vi "WLAN_be_EVMvi.vi"(5 "Function":T1, 7 "setPower":i32, 8 "error in":errorcluster, 11 "VISA IN":refnum<visa-resource-name>="IQGIG") -> (0 "error out":errorcluster, 1 "EVM":dbl, 2 "Power":dbl, 3 "IDN":string)   [LabVIEW 2023, in "LitePoints.lvlib"]
uses:
  LitePoints.lvlib
  CTL/LitePoint_EVM.ctl
panel:
  out "forREF_PW":string
  out "Response_EVM":string
  out "Response_PW":string
  out "VSA_Ref?":string
  out "VSA?":string
  out "Clean Buffer?":string
  out "setPower?":string
  # "IQgig-5G : TCPIP0::192.168.100.254::hislip0::INSTR"
  # "IQxel-MX : TCPIP0::192.168.100.253::hislip0::INSTR"
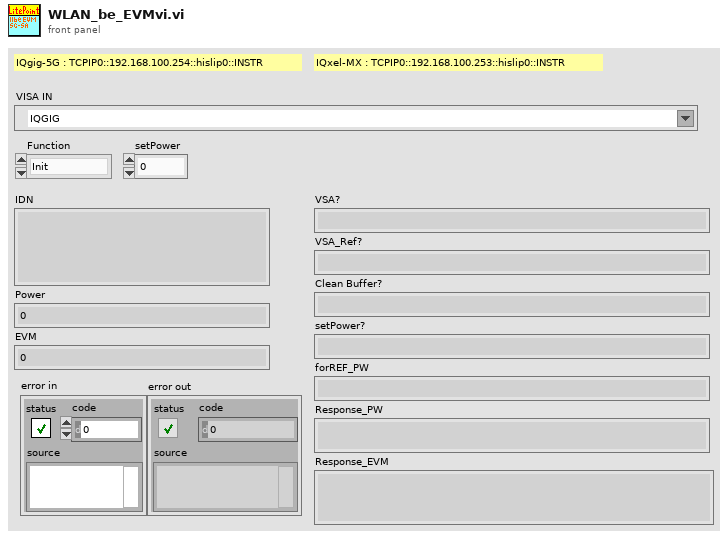
[diagram p1: front panel]
types:
  T1 = typedef "LitePoint_EVM.ctl" = enum16{"Init", "Close", "set_SG", "set_SA", "get_EVM", "byPass", "getPower"}
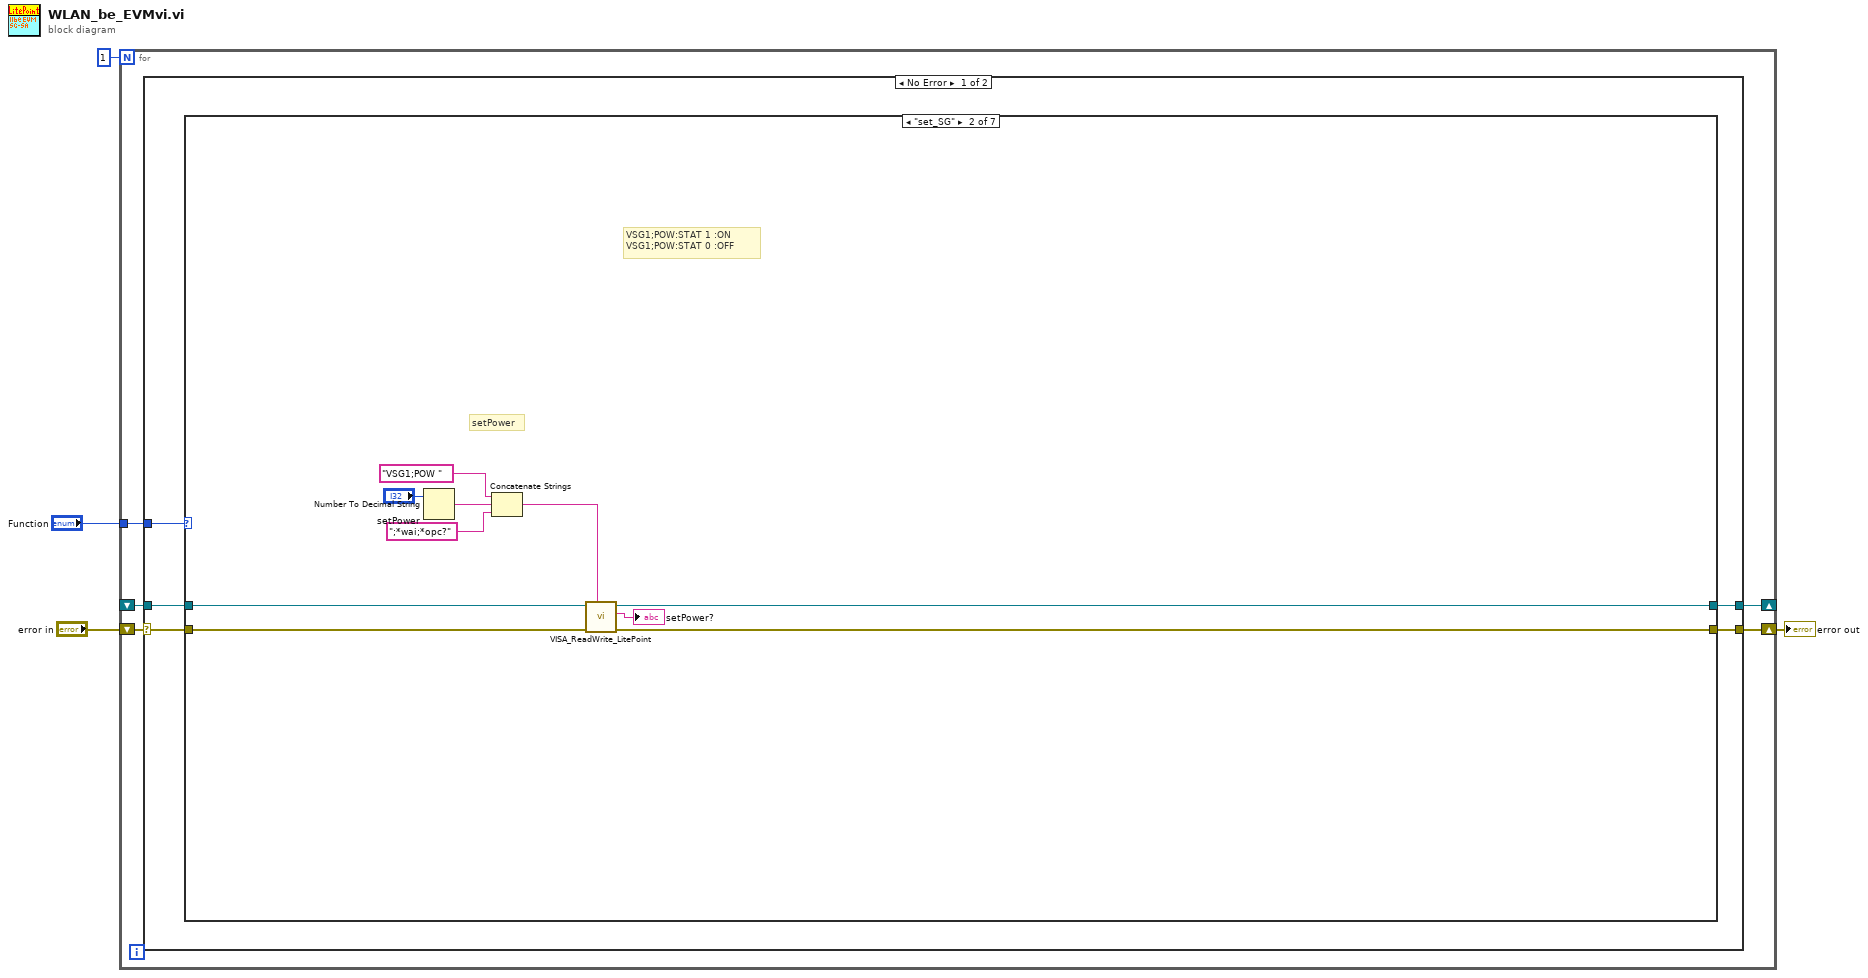
[diagram p0: block diagram]
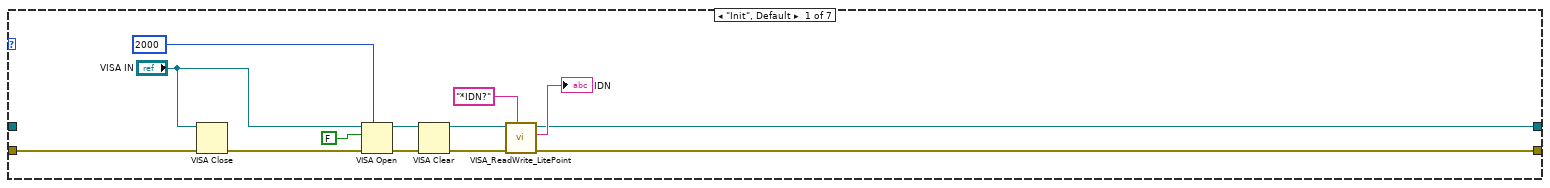
[diagram p2: hidden frame]
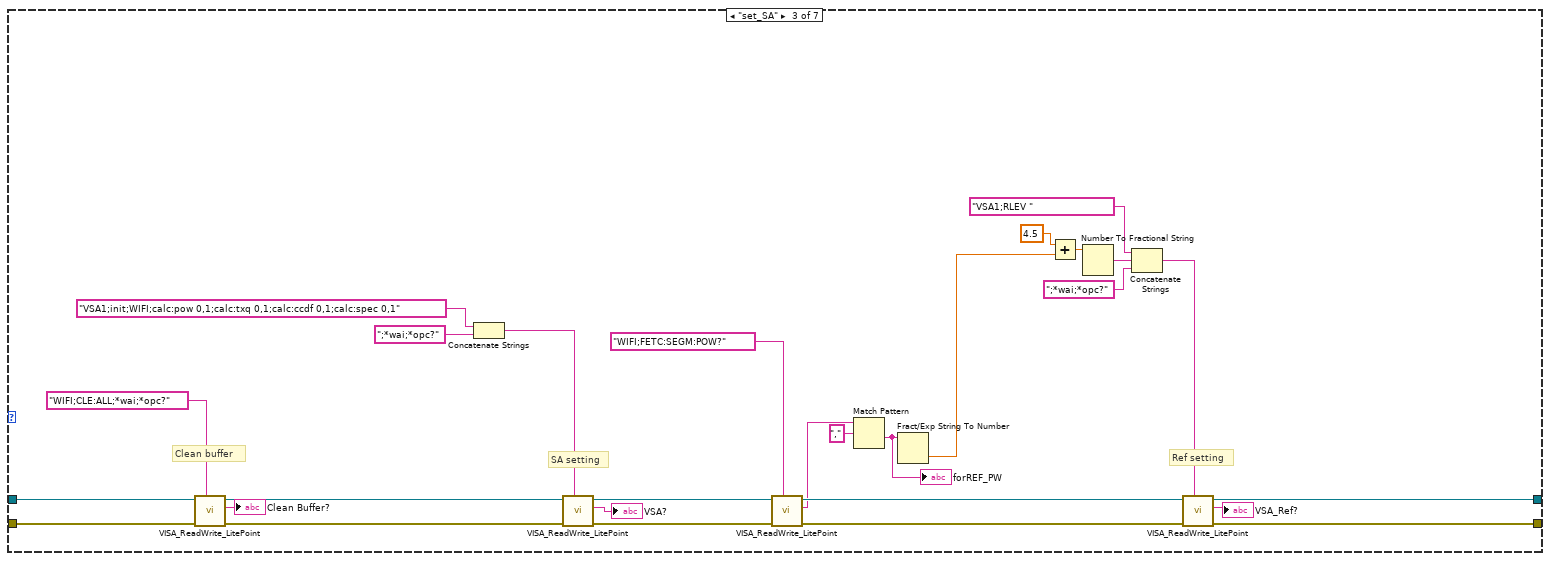
[diagram p3: hidden frame]
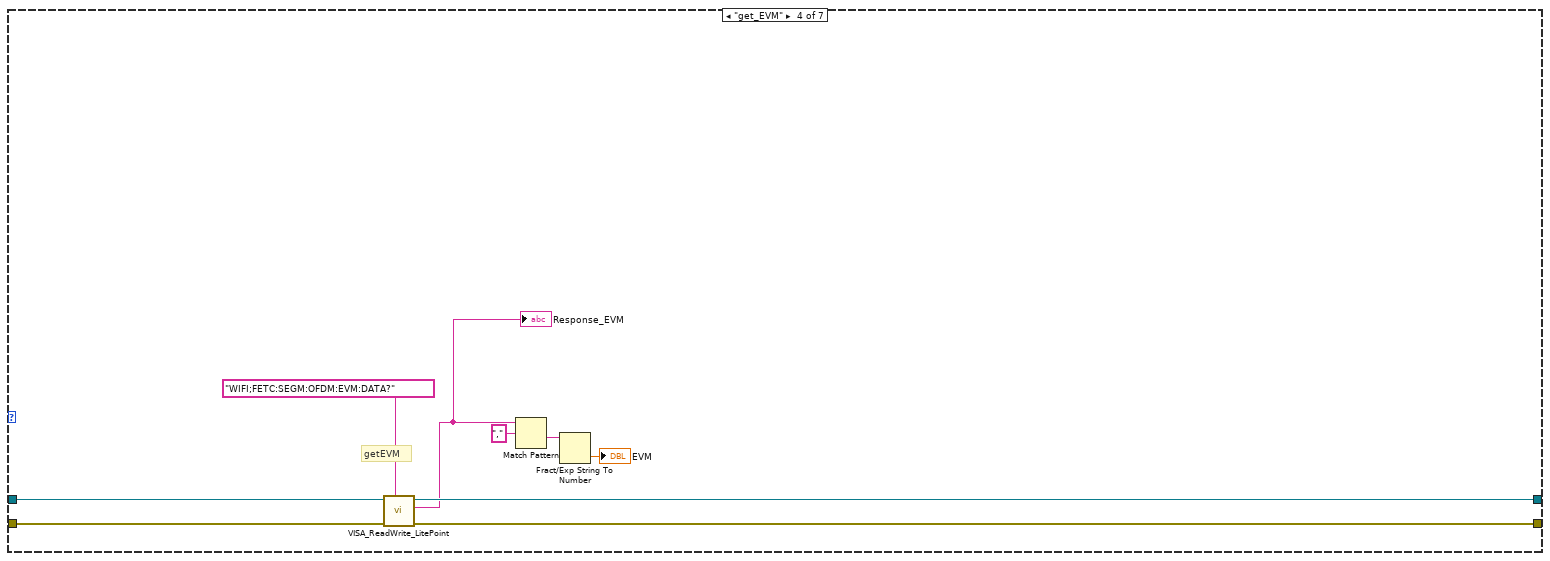
[diagram p4: hidden frame]
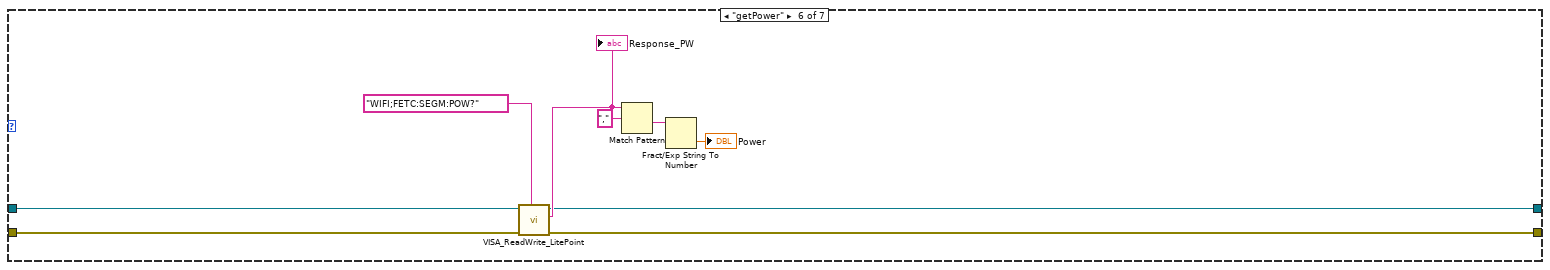
[diagram p6: hidden frame]
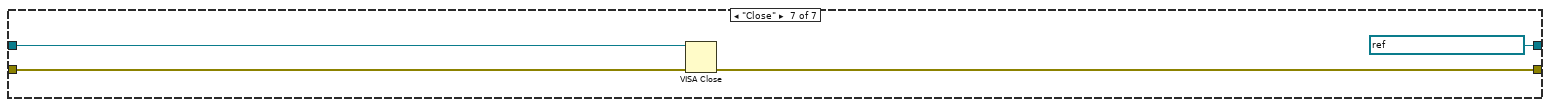
[diagram p7: hidden frame]
diagram:
  n1 = for {
    N: 1 -> [_]
    tunnel: "Function" -> [w7]
    shift-right: [w8] -> w3
    shift-left: "error in" -> [w9]
    shift-right: [w5] -> _
    shift-left: _ -> [w6]
    n2 = case shown="No Error" w9 {
      selector: w9 -> [w13 w91]
      tunnel: [w12 w91] -> w8
      tunnel: w7 -> [w14 _]
      tunnel: w6 -> [w11 w90]
      tunnel: [w10 w90] -> w5
      frame No Error {
        n3 = case shown="\"set_SG\"" w14 {
          tunnel: [w22 w28 w51 w71 w76 w84 w89] -> w12
          tunnel: w13 -> [w17 w32 w65 w74 w76 w85 w88]
          tunnel: w11 -> [_ w33 w64 w73 w75 w79 w87]
          tunnel: [w18 w29 w52 w70 w75 w78 refnum<visa-resource-name> refnum ("VISA out")] -> w10
          frame "Init", Default {
            n4 = VISA Close(VISA resource name="VISA IN", error in (no error)=w17) -> (error out=w16:errorcluster)
            n5 = VISA Open(timeout (0)=u32 2000 ("VISA Open timeout (0)"), duplicate session (F)=FALSE, error in (no error)=w16, VISA resource name="VISA IN") -> (VISA resource name=w24:refnum<visa-resource-name>, error out=w25:errorcluster)  [unwired: 1 in]
            n6 = VISA Clear(VISA resource name=w24, error in (no error)=w25) -> (VISA resource name out=w21:refnum<visa-resource-name>, error out=w23:errorcluster)
            n7 = call "VISA_ReadWrite_LitePoint.vi"("VISA_CMD"="*IDN?", "error in"=w23, "VISA in"=w21) -> ("error out"=w22:errorcluster, "Response"=→"IDN":string, "VISA out"=w18:refnum<visa-resource-name>)  [unwired: 6 in]
          }
          frame "set_SG" {
            # "VSG1;POW:STAT 1 :ON\nVSG1;POW:STAT 0 :OFF"
            # "setPower"
            n8 = Number To Decimal String(number="setPower") -> (decimal integer string=w37:string)  [unwired: 1 in]
            n9 = Concatenate Strings("VSG1;POW " ("write buffer"), w37, ";*wai;*opc?" ("write buffer")) -> (w31:string)
            n10 = call "VISA_ReadWrite_LitePoint.vi"("VISA_CMD"=w31, "error in"=w32, "VISA in"=w33) -> ("error out"=w28:errorcluster, "Response"=→"setPower?":string, "VISA out"=w29:refnum<visa-resource-name>)  [unwired: 6 in]
          }
          frame "set_SA" {
            # "Ref setting"
            # "SA setting"
            # "Clean buffer"
            n11 = call "VISA_ReadWrite_LitePoint.vi"("VISA_CMD"="WIFI;CLE:ALL;*wai;*opc?" ("write buffer"), "error in"=w65, "VISA in"=w64) -> ("error out"=w57:errorcluster, "Response"=→"Clean Buffer?":string, "VISA out"=w58:refnum<visa-resource-name>)  [unwired: 6 in]
            n12 = Concatenate Strings("VSA1;init;WIFI;calc:pow 0,1;calc:txq 0,1;calc:ccdf 0,1;calc:spec 0,1" ("write buffer"), ";*wai;*opc?" ("write buffer")) -> (w59:string)
            n13 = call "VISA_ReadWrite_LitePoint.vi"("VISA_CMD"=w59, "error in"=w57, "VISA in"=w58) -> ("error out"=w46:errorcluster, "Response"=→"VSA?":string, "VISA out"=w44:refnum<visa-resource-name>)  [unwired: 6 in]
            n14 = call "VISA_ReadWrite_LitePoint.vi"("VISA_CMD"="WIFI;FETC:SEGM:POW?" ("write buffer"), "error in"=w46, "VISA in"=w44) -> ("error out"=w45:errorcluster, "Response"=w39:string, "VISA out"=w43:refnum<visa-resource-name>)  [unwired: 6 in]
            n15 = Match Pattern(string=w39, regular expression=",") -> (after substring=w40:string)  [unwired: 1 in, 3 out]
            "forREF_PW" <- w40
            n16 = Fract/Exp String To Number(string=w40) -> (number=w38:dbl)  [unwired: 3 in, 1 out]
            n17 = Add(x=4.5, y=w38) -> (x+y=w47:dbl)
            n18 = Number To Fractional String(number=w47) -> (F-format string=w53:string)  [unwired: 3 in]
            n19 = Concatenate Strings("VSA1;RLEV " ("write buffer"), w53, ";*wai;*opc?" ("write buffer")) -> (w50:string)
            n20 = call "VISA_ReadWrite_LitePoint.vi"("VISA_CMD"=w50, "error in"=w45, "VISA in"=w43) -> ("error out"=w51:errorcluster, "Response"=→"VSA_Ref?":string, "VISA out"=w52:refnum<visa-resource-name>)  [unwired: 6 in]
          }
          frame "get_EVM" {
            # "getEVM"
            n21 = call "VISA_ReadWrite_LitePoint.vi"("VISA_CMD"="WIFI;FETC:SEGM:OFDM:EVM:DATA?" ("write buffer"), "error in"=w74, "VISA in"=w73) -> ("error out"=w71:errorcluster, "Response"=w68:string, "VISA out"=w70:refnum<visa-resource-name>)  [unwired: 6 in]
            "Response_EVM" <- w68
            n22 = Match Pattern(string=w68, regular expression=",") -> (after substring=w67:string)  [unwired: 1 in, 3 out]
            n23 = Fract/Exp String To Number(string=w67) -> (number=→"EVM":dbl)  [unwired: 3 in, 1 out]
          }
          frame "byPass" {
          }
          frame "getPower" {
            n24 = call "VISA_ReadWrite_LitePoint.vi"("VISA_CMD"="WIFI;FETC:SEGM:POW?" ("write buffer"), "error in"=w85, "VISA in"=w79) -> ("error out"=w84:errorcluster, "Response"=w80:string, "VISA out"=w78:refnum<visa-resource-name>)  [unwired: 6 in]
            "Response_PW" <- w80
            n25 = Match Pattern(string=w80, regular expression=",") -> (after substring=w81:string)  [unwired: 1 in, 3 out]
            n26 = Fract/Exp String To Number(string=w81) -> (number=→"Power":dbl)  [unwired: 3 in, 1 out]
          }
          frame "Close" {
            n27 = VISA Close(VISA resource name=w87, error in (no error)=w88) -> (error out=w89:errorcluster)
          }
        }
      }
      frame Error {
      }
    }
  }
  "error out" <- w3
